vi "dZj(r,theta).vi"(4 "error in (no error)":errorcluster, 5 "theta":dbl, 6 "r":dbl, 7 "j (1)":i32=1) -> (0 "error out":errorcluster, 3 "dZj(r,theta)":T1)   [LabVIEW 2013, in "Zernike Polynome.lvlib"]
doc: "This VI calculates the derivative of Zj(r,theta) in x- and y-directions."
uses:
  Zernike Polynome.lvlib
  dZj(r,theta).ctl
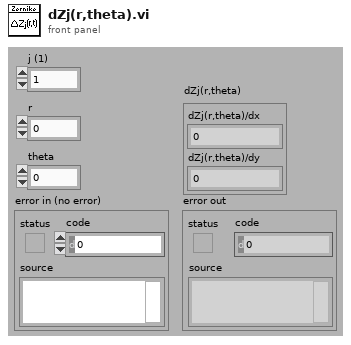
[diagram p1: front panel]
types:
  T1 = typedef "Zernike Polynome.lvlib/dZj(r,theta).ctl" = cluster{"dZj(r,theta)/dx":dbl, "dZj(r,theta)/dy":dbl}
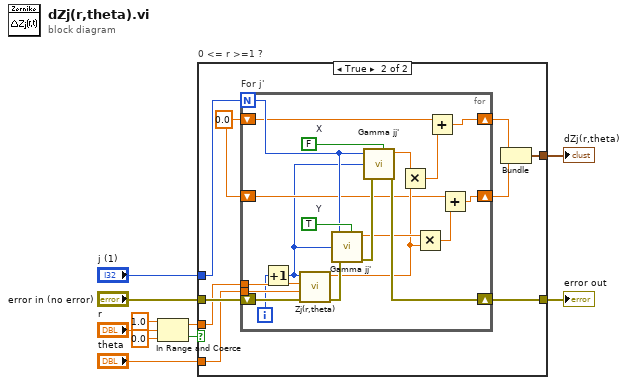
[diagram p0: block diagram]
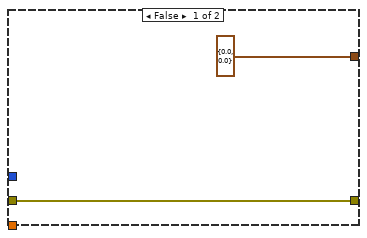
[diagram p2: hidden frame]
diagram:
  n1 = In Range and Coerce(upper limit=1.0, x="r", lower limit=0.0) -> (coerced(x)=w6:dbl, In Range?=w3:bool)
  n2 = case "0 <= r >=1 ?" shown="True" w3 {
    tunnel: "error in (no error)" -> [w12 w21]
    tunnel: [cluster{dbl, dbl} {0.0, 0.0} w13] -> w1
    tunnel: "j (1)" -> [_ w17]
    tunnel: "theta" -> [_ w18]
    tunnel: w6 -> [_ w19]
    tunnel: [w12 w20] -> w2
    frame False {
    }
    frame True {
      w16 = 0.0
      n3 = for "For j'" {
        N: w17 -> [w31]
        tunnel: w19 -> [w40]
        tunnel: w18 -> [w39]
        shift-right: [w33] -> w20
        shift-left: w21 -> [w41]
        shift-right: [w27] -> w15
        shift-left: w16 -> [w26]
        shift-right: [w24] -> w14
        shift-left: w16 -> [w23]
        i -> [w38]
        w35 = TRUE  # Y
        w36 = FALSE  # X
        n4 = Increment(x=w38) -> (x+1=w22:i32)
        n5 = call "Zj(r,theta).vi"("error in (no error)"=w41, "theta"=w39, "r"=w40, "j (1)"=w22) -> ("error out"=w34:errorcluster, "Zj(r,theta)"=w29:dbl)  [unwired: 2 out]
        n6 = call "Gamma jj'.vi"("X/Y"=w35, "error in (no error)"=w34, "j' (1)"=w22, "j (1)"=w31) -> ("error out"=w37:errorcluster, "Gamma Magnitude"=w30:dbl)  [unwired: 2 out]
        n7 = call "Gamma jj'.vi"("X/Y"=w36, "error in (no error)"=w37, "j' (1)"=w22, "j (1)"=w31) -> ("error out"=w33:errorcluster, "Gamma Magnitude"=w32:dbl)  [unwired: 2 out]
        n8 = Multiply(x=w32, y=w29) -> (x*y=w28:dbl)
        n9 = Multiply(x=w30, y=w29) -> (x*y=w25:dbl)
        n10 = Add(x=w26, y=w28) -> (x+y=w27:dbl)
        n11 = Add(x=w23, y=w25) -> (x+y=w24:dbl)
      }
      n12 = Bundle(w15, w14) -> (w13:cluster{dbl, dbl})  [unwired: 1 in]
    }
  }
  "error out" <- w2
  "dZj(r,theta)" <- w1
